vi "GetRfsaSession.vi"(8 "error in (no error)":errorcluster, 11 "Instrument Handle In":refnum<k21>) -> (0 "error out":errorcluster, 2 "NI RFSA Session":refnum<k15>, 3 "Instrument Handle Out":refnum<k21>)   [LabVIEW 2019]
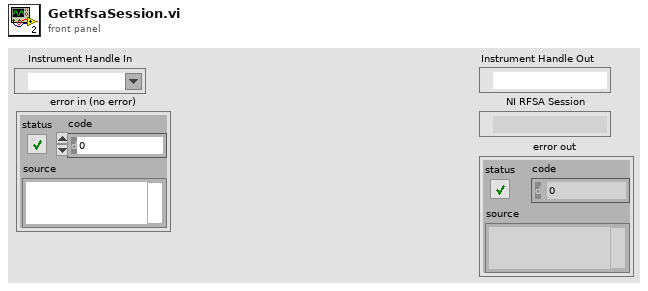
[diagram p1: front panel]
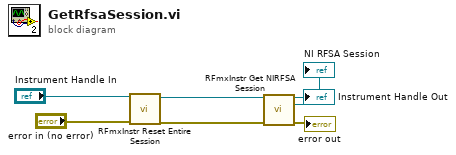
[diagram p0: block diagram]
diagram:
  n1 = call <vilib>:"RFmxInstr Reset Entire Session.vi"("Instrument Handle In"="Instrument Handle In", "error in (no error)"="error in (no error)") -> ("Instrument Handle Out"=w7:refnum<k21>, "error out"=w6:errorcluster)  [unwired: 12 in]
  n2 = call <vilib>:"RFmxInstr Get NIRFSA Session.vi"("Instrument Handle In"=w7, "error in (no error)"=w6) -> ("Instrument Handle Out"=→"Instrument Handle Out":refnum<k21>, "NI RFSA Session"=→"NI RFSA Session":refnum<k15>, "error out"=→"error out":errorcluster)  [unwired: 11 in]
